vi "initialize.vi"(8 "error in":errorcluster, 11 "Data Cluster":variant) -> (0 "error out":errorcluster, 2 "channel names":string[](array[string]), 3 "stream custom cluster":refnum<class "stream_custom_cluster.lvclass">)   [LabVIEW 2020, in "stream_custom_cluster.lvclass"]
doc: "Sets up backend buffers and analyzes the cluster structure.\nThis function does not send or capture data.\nPerforms datatype validation and buffer setup.\n\nCluster Element Requirements\nClusters must contain only the following data types:\n- Signed Integers (I8, I16, I32, I64)\n- Unsigned Integers (U8, U16, U32, U64)\n- Singles (SGL)\n- Doubles (DBL)\n- Booleans\n- Strings\n- Nested Clusters\nNested clusters are supported and can contain any combination of the above data types.\nThe cluster and all elements must be named.\n\nSee `Streaming Cluster Data` example for useage notes."
uses:
  stream_custom_cluster.lvclass
  private data.ctl
  <userlib>/_OpenG.lib/lvdata/lvdata.llb/Type Descriptor Enumeration__ogtk.ctl
  stream_custom_cluster.lvclass/stream_custom_cluster.ctl
  <userlib>/_OpenG.lib/lvdata/lvdata.llb/openg_variant.lvlib
  <vilib>/Utility/Data Type/NI_Data Type.lvlib
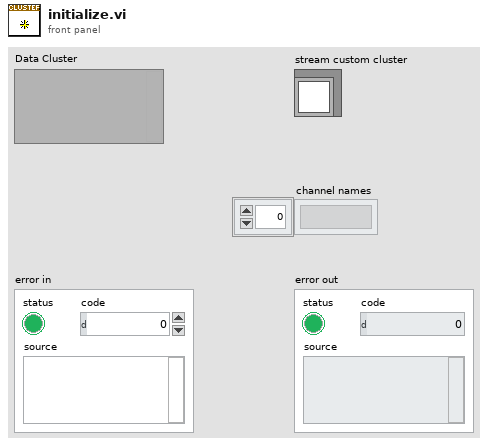
[diagram p1: front panel]
types:
  T1 = cluster{"timestamp":cluster{"seconds":i32, "nanos":i32}, "value":variant}
  T2 = typedef "openg_variant.lvlib/Type Descriptor Enumeration__ogtk.ctl" = enum8{"<Null>", "I8", "I16", "I32", "I64", "U8", "U16", "U32", "U64", "SGL", "DBL", "EXT", "CSG", "CDB", "CXT", "0x0F", "0x10", "0x11", "0x12", "0x13", "0x14", "Enum U8", "Enum U16", "Enum U32", "Enum U64", "SGL PQ", "DBL PQ", "EXT PQ", "CSG PQ", "CDB PQ", "CXT PQ", "0x1F", "0x20", "Boolean", "0x22", "0x23", "0x24", "0x25", "0x26", "0x27", "0x28", "0x29", "0x2A", "0x2B", "0x2C", "0x2D", "0x2E", "0x2F", "String", "0x31", "Path", "Pict", "0x34", "0x35", "0x36", "DAQ", "0x38", "0x39", "0x3A", "0x3B", "0x3C", "0x3D", "0x3E", "0x3F", "Array", "0x41", "0x42", "0x43", "0x44", "0x45", "0x46", "0x47", "0x48", "0x49", "0x4A", "0x4B", "0x4C", "0x4D", "0x4E", "0x4F", "Cluster", "0x51", "0x52", "Variant", "Waveform", "0x55", "0x56", "0x57", "0x58", "0x59", "0x5A", "0x5B", "0x5C", "0x5D", "0x5E", "Fixed Point", "0x60", "0x61", "0x62", "0x63", "0x64", "0x65", "0x66", "0x67", "0x68", "0x69", "0x6A", "0x6B", "0x6C", "0x6D", "0x6E", "0x6F", "Refnum", "0x71", "0x72", "Set Collection", "Map Collection"}
  T3 = typedef "stream_custom_cluster.lvclass/private data.ctl" = cluster{"type":T2[], "channel names":string[], "data":refnum<queue>[], "cluster element types":variant[]}
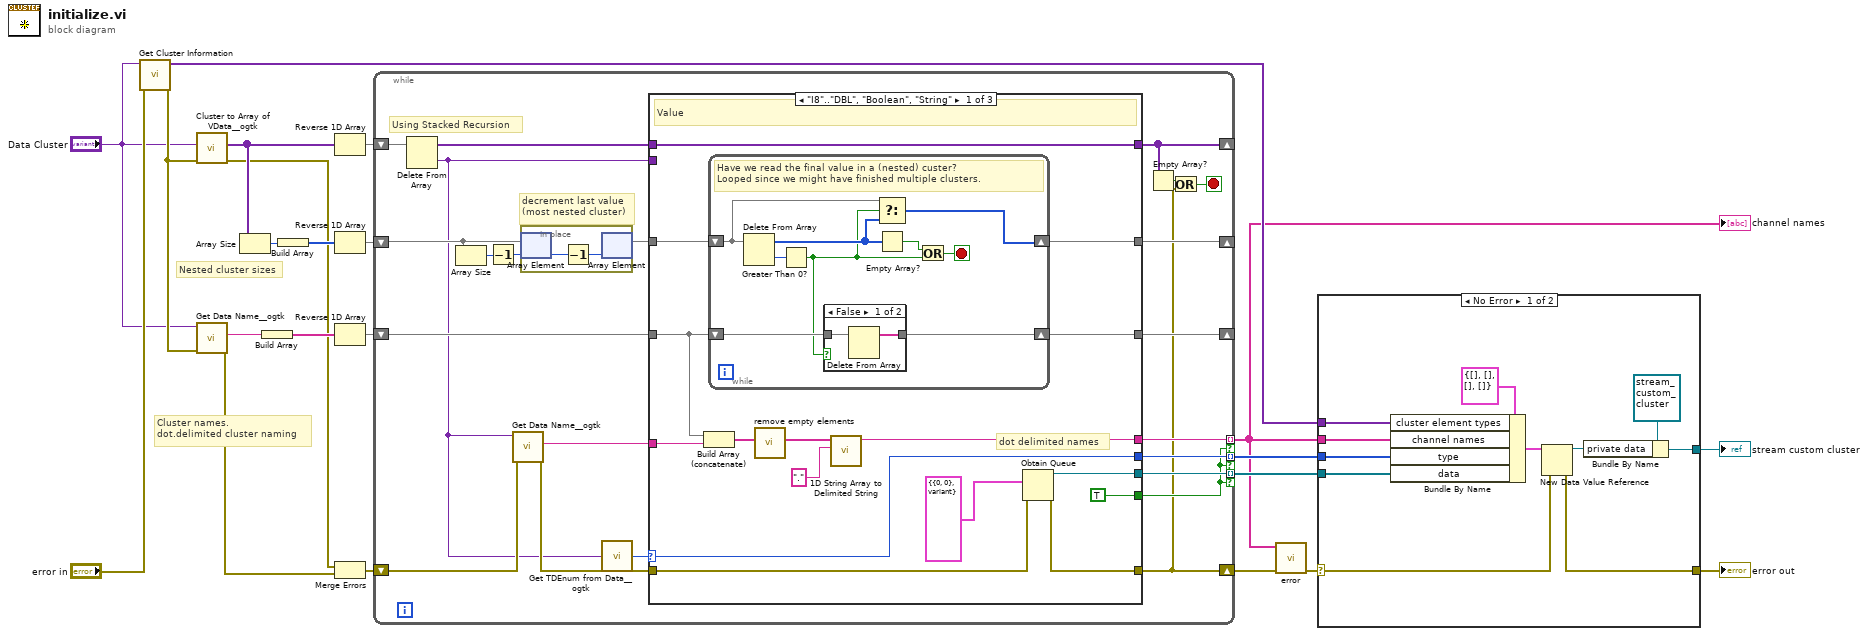
[diagram p0: block diagram]
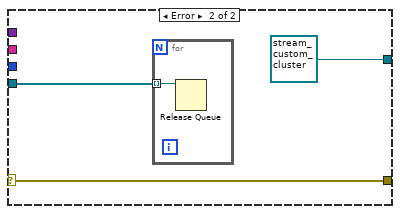
[diagram p2: hidden frame]
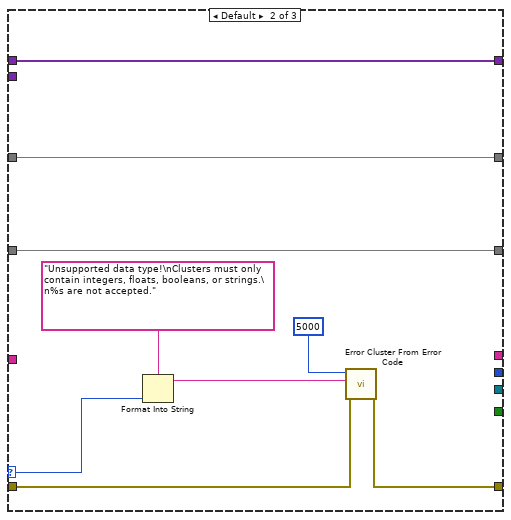
[diagram p4: hidden frame]
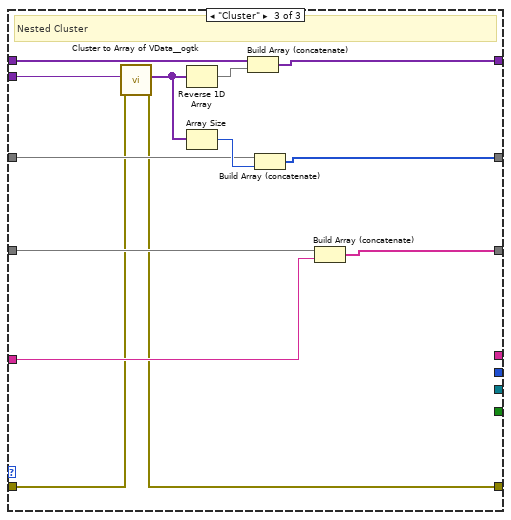
[diagram p5: hidden frame]
diagram:
  # "Nested cluster sizes"
  # "Cluster names.\ndot.delimited cluster naming"
  n1 = call <vilib>:"Get Cluster Information.vi"("error in (no error)"="error in", "variant"="Data Cluster") -> ("error out"=w5:errorcluster, "cluster elements"=w7:variant[])  [unwired: 8 in]
  n2 = call <userlib>:"Cluster to Array of VData__ogtk.vi"("error in (no error)"=w5, "Cluster"="Data Cluster") -> ("error out"=w14:errorcluster, "Array of VData"=w22:variant[])  [unwired: 8 in]
  n3 = call <userlib>:"Get Data Name__ogtk.vi"("error in (no error)"=w5, "Data"="Data Cluster") -> ("error out"=w13:errorcluster, "Data Name"=w21:string)  [unwired: 7 in, 1 out]
  n4 = Array Size(array=w22) -> (size(s)=w20:i32)
  n5 = Build Array(w21) -> (w18:string[])
  n6 = Build Array(w20) -> (w19:i32[])
  n7 = Reverse 1D Array(array=w22) -> (reversed array=w17:variant[])
  n8 = Reverse 1D Array(array=w19) -> (reversed array=w16:i32[])
  n9 = Reverse 1D Array(array=w18) -> (reversed array=w15:string[])
  n10 = Merge Errors(w14, w13) -> (w12:errorcluster)
  n11 = while {
    shift-right: [w39] -> _
    shift-left: w17 -> [w44]
    shift-right: [w41] -> _
    shift-left: w15 -> [w40]
    shift-right: [w38] -> _
    shift-left: w16 -> [w32]
    shift-right: [w24] -> w3
    shift-left: w12 -> [w34]
    tunnel: [w28] -> w1 mode=indexing if=w25
    tunnel: [w27] -> w9 mode=indexing if=w25
    tunnel: [w26] -> w8 mode=indexing if=w25
    stop <- w36 stop-if-true
    # "Using Stacked Recursion"
    # "decrement last value\n(most nested cluster)"
    n12 = Delete From Array(array=w44) -> (deleted portion=w23:variant, array with subset deleted=w42:variant[])  [unwired: 2 in]
    n13 = Array Size(array=w32) -> (size(s)=w30:i32)
    n14 = Decrement(x=w30) -> (x-1=w29:i32)
    n15 = call <userlib>:"Get Data Name__ogtk.vi"("error in (no error)"=w34, "Data"=w23) -> ("error out"=w33:errorcluster, "Data Name"=w35:string)  [unwired: 7 in, 1 out]
    n16 = in-place {
      n17 = in-place-array #1(w32, w29) -> (w46:i32)
      n18 = Decrement(x=w46) -> (x-1=w45:i32)
      n19 = in-place-array #1(w45) -> (w31:i32[])  [unwired: 1 out]
    }
    n20 = call <userlib>:"Get TDEnum from Data__ogtk.vi"("Data"=w23) -> ("Type Descriptor Enumeration"=w43:T2)  [unwired: 4 in]
    n21 = case shown="\"I8\"..\"DBL\", \"Boolean\", \"String\"" w43 {
      selector: w43 -> [w57 w81 _]
      tunnel: w23 -> [_ _ w87]
      tunnel: [w62 w77 w94] -> w39
      tunnel: w42 -> [w62 w77 w95]
      tunnel: [w59 w75 w88] -> w41
      tunnel: w40 -> [w50 w75 w93]
      tunnel: w35 -> [w58 _ w92]
      tunnel: [w60 w76 w90] -> w38
      tunnel: w31 -> [w61 w76 w89]
      tunnel: w33 -> [w53 w80 w86]
      tunnel: [w54 _ _] -> w28
      tunnel: [w57 _ _] -> w27
      tunnel: [w56 _ _] -> w26
      tunnel: [TRUE _ _] -> w25
      tunnel: [w52 w79 w84] -> w24
      frame "I8".."DBL", "Boolean", "String" {
        # "dot delimited names"
        # "Value"
        n22 = Build Array (concatenate)(w50, w58) -> (w49:string[])
        n23 = while {
          shift-right: [w70] -> w60
          shift-left: w61 -> [w71]
          shift-right: [w64] -> w59
          shift-left: w50 -> [w66]
          stop <- w67 stop-if-true
          # "Have we read the final value in a (nested) custer?\nLooped since we might have finished multiple clusters."
          n24 = Delete From Array(array=w71) -> (deleted portion=w63:i32, array with subset deleted=w69:i32[])  [unwired: 2 in]
          n25 = Greater Than 0?(x=w63) -> (x > 0?=w65:bool)
          n26 = case shown="False" w65 {
            tunnel: w66 -> [w73 w74]
            tunnel: [w72 w74] -> w64
            frame False {
              n27 = Delete From Array(array=w73) -> (array with subset deleted=w72:string[])  [unwired: 2 in, 1 out]
            }
            frame True {
            }
          }
          n28 = Select(t=w71, s=w65, f=w69) -> (s? t:f=w70:i32[])
          n29 = Empty Array?(array=w69) -> (empty?=w68:bool)
          n30 = Or(x=w68, y=w65) -> (x .or. y?=w67:bool)
        }
        n31 = call "remove empty elements.vi"("array in"=w49) -> ("array without blanks out"=w48:string[])  [unwired: 10 in]
        n32 = call <vilib>:"1D String Array to Delimited String.vi"("delimiter"=".", "string array"=w48) -> ("delimited string"=w54:string)  [unwired: 9 in]
        n33 = Obtain Queue(element data type=T1 {"timestamp"={"seconds"=0, "nanos"=0}, "value"=variant} ("value"), error in (no error)=w53) -> (queue out=w56:refnum<queue>, error out=w52:errorcluster)  [unwired: 3 in, 1 out]
      }
      frame Default {
        n34 = Format Into String(format string="Unsupported data type!\nClusters must only contain integers, floats, booleans, or strings.\n%s are not accepted." ("message"), w81) -> (resulting string=w82:string)  [unwired: 2 in, 1 out]
        n35 = call <vilib>:"Error Cluster From Error Code.vi"("error in (no error)"=w80, "error message (\"\")"=w82, "error code (0)"=5000) -> ("error out"=w79:errorcluster)  [unwired: 6 in]
      }
      frame "Cluster" {
        # "Nested Cluster"
        n36 = call <userlib>:"Cluster to Array of VData__ogtk.vi"("error in (no error)"=w86, "Cluster"=w87) -> ("error out"=w84:errorcluster, "Array of VData"=w85:variant[])  [unwired: 8 in]
        n37 = Reverse 1D Array(array=w85) -> (reversed array=w96:variant[])
        n38 = Array Size(array=w85) -> (size(s)=w91:i32)
        n39 = Build Array (concatenate)(w95, w96) -> (w94:variant[])
        n40 = Build Array (concatenate)(w89, w91) -> (w90:i32[])
        n41 = Build Array (concatenate)(w93, w92) -> (w88:string[])
      }
    }
    n42 = Empty Array?(array=w39) -> (empty?=w37:bool)
    n43 = Or(x=w37, y=w24) -> (x .or. y?=w36:bool)
  }
  "channel names" <- w1
  n44 = call "error.vi"("error in"=w3, "channel names"=w1) -> ("error out"=w2:errorcluster)  [unwired: 9 in]
  n45 = case shown="No Error" w2 {
    selector: w2 -> [w107 w110]
    tunnel: [w106 w110] -> w11
    tunnel: [w104 refnum<class "stream_custom_cluster.lvclass"> refnum ("stream_custom_cluster out")] -> w10
    tunnel: w1 -> [w103 _]
    tunnel: w9 -> [w102 _]
    tunnel: w8 -> [w101 w108]
    tunnel: w7 -> [w97 _]
    frame No Error {
      n46 = Bundle By Name(cluster=T3 {"type"=[], "channel names"=[], "data"=[], "cluster element types"=[]} ("Cluster"), "cluster element types"=w97, "channel names"=w103, "type"=w102, "data"=w101) -> (w100:T3)
      n47 = New Data Value Reference(data value=w100, error in=w107) -> (data value reference=w98:refnum<data-value>, error out=w106:errorcluster)
      n48 = Bundle By Name(cluster=refnum<class "stream_custom_cluster.lvclass"> refnum ("stream_custom_cluster out"), "private data"=w98) -> (w104:refnum<class "stream_custom_cluster.lvclass">)
    }
    frame Error {
      n49 = for {
        tunnel: w108 -> [w111] mode=indexing
        n50 = Release Queue(queue=w111) -> ()  [unwired: 2 in, 3 out]
      }
    }
  }
  "stream custom cluster" <- w10
  "error out" <- w11
